vi "NT Client_NoDS.vi"(6 "Update Time":i32=100, 9 "Client Name":string="Dashboard", 11 "TEAM":u32=4150) -> (0 "error out":errorcluster={"status"=FALSE, "code"=-1, "source"=""})   [LabVIEW 2025]
doc: "Place this VI in the Dashboard or other client applications. Provide the robot IP address so that it can know where to find the server.\n\nYou normally want the restart option to be true, but if you have your own restart strategy, you can disable it. Tracing is useful when debugging. Similarly, the disconnect timout may need to be raised if setting breakpoints. The user event ref will publish the client activities so that other elements of the dashboard are notified when packets are processed."
uses:
  <vilib>/Rock Robotics/Network Tables/NT Globals.vi
  FRC_NetworkTablesLV.dll
  ntcoreffi.dll
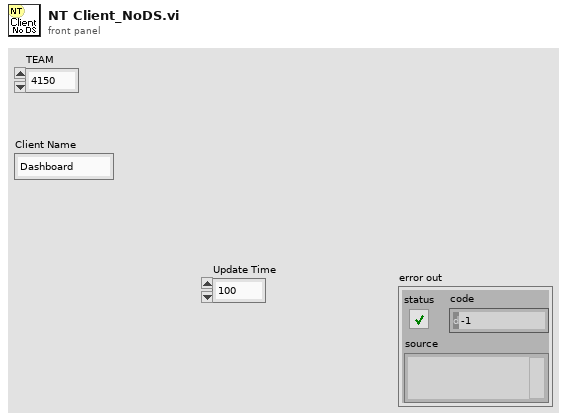
[diagram p1: front panel]
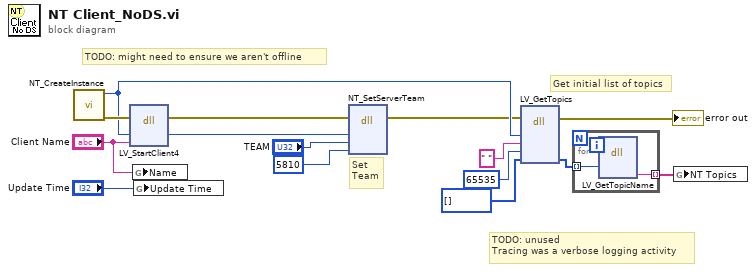
[diagram p0: block diagram]
diagram:
  # "Set \nTeam"
  # "Get initial list of topics"
  # "TODO: might need to ensure we aren't offline"
  # "TODO: unused\nTracing was a verbose logging activity"
  n1 = call <vilib>:"NT_CreateInstance.vi"() -> ("error out"=w14:errorcluster, "InstanceHandle"=w12:u64)  [unwired: 10 in]
  n2 = dll-call lib="FRC_NetworkTablesLV.*" fn="LV_StartClient4"(error in=w14, "InstHandle"=w12, "identity"="Client Name") -> (error out=w6:errorcluster, "InstHandle"=w5:u64)  [unwired: 4 in, 1 out]
  n3 = global write "NT Globals.vi" "Name"("Client Name") -> ()
  n4 = global write "NT Globals.vi" "Update Time"("Update Time") -> ()
  n5 = dll-call lib="ntcoreffi.*" fn="NT_SetServerTeam"(error in=w6, "inst"=w5, "TEAM"="TEAM", "port"=u32 5810) -> (error out=w3:errorcluster)  [unwired: 6 in, 1 out]
  n6 = dll-call lib="FRC_NetworkTablesLV.*" fn="LV_GetTopics"(error in=w3, "inst"=w12, "prefix"=" ", "typeMask"=u32 65535, "topicsArray"=u32[] []) -> (error out=→"error out":errorcluster, "topicsArray"=w9:u32[])  [unwired: 6 in, 1 out]
  n7 = for {
    tunnel: [w16] -> w10 mode=indexing
    tunnel: w9 -> [w17] mode=indexing
    n8 = dll-call lib="FRC_NetworkTablesLV.*" fn="LV_GetTopicName"("topic"=w17) -> ("name"=w16:string)  [unwired: 6 in, 2 out]
  }
  n9 = global write "NT Globals.vi" "NT Topics"(w10) -> ()
